vi "leybold.vi"() -> ()   [LabVIEW 2023]
panel:
  in  "RS232":bool
  in  "recipes":bool
  out "Time":timestamp format="%<%H:%M:%S\n%x>T"
  out "Timer end":timestamp format="%<%H:%M:%S>T"
  in  "P3":bool
  in  "P2":bool
  in  "Presets":bool
  out "PR4000":string
  in  "TimerOn":bool
  in  "Matchbox mode":bool
  in  "Timer":bool
  in  "GAS Boost":bool
  in  "-100":bool
  in  "-10":bool
  in  "-1":bool
  in  "+1":bool
  in  "+10":bool
  in  "Gas":bool
  in  "O2 (SCCM)":bool
  in  "Ar (SCCM)":bool
  out "DC Bias (V)":i16
  in  "+100":bool
  in  "Stop":bool
  out "read buffer":string
  out "PFG600":string
  in  "RF Source":bool
  in  "CT":bool
  in  "CL":bool
  in  "FWD Power (W)":bool=TRUE
  out "REF Power (W)":i16
  # "GENERATOR"
  # "MFC"
  # "TIMER"
  # "DEBUG"
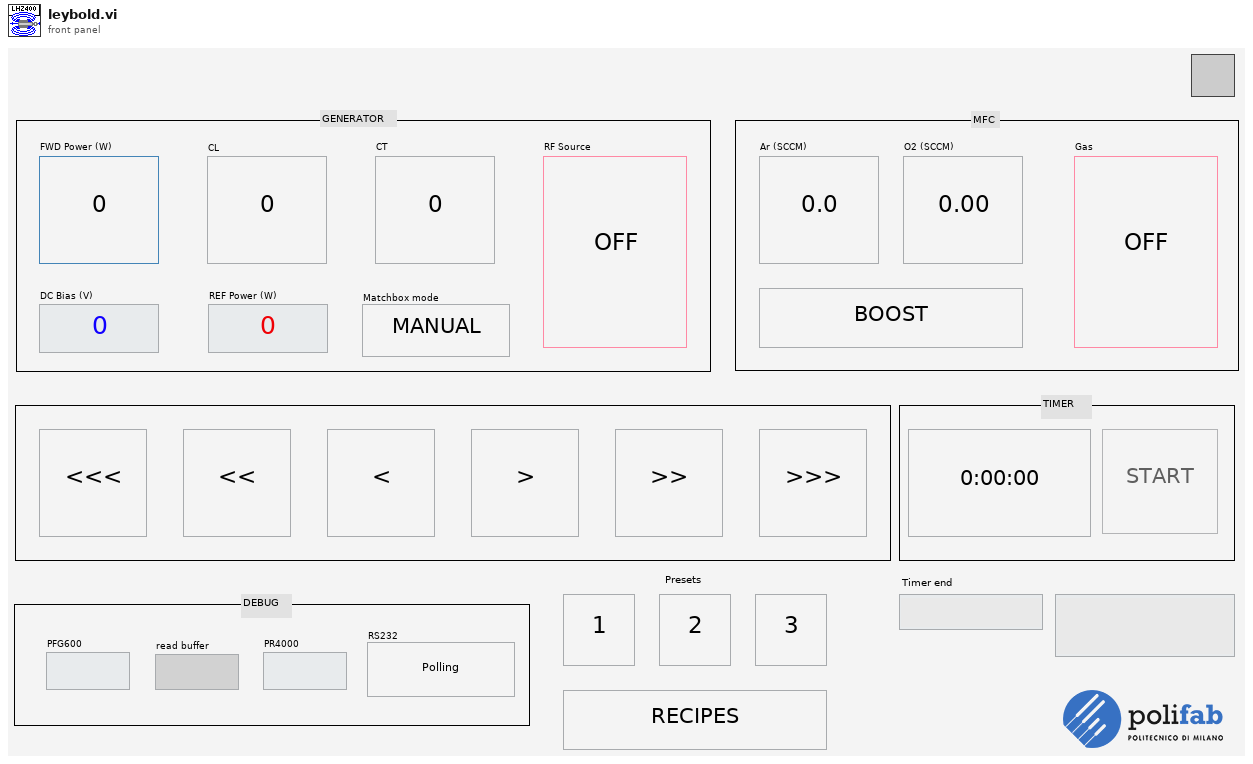
[diagram p1: front panel]
types:
  T1 = enum8{"Enabled", "Disabled", "Disabled and Grayed Out"}
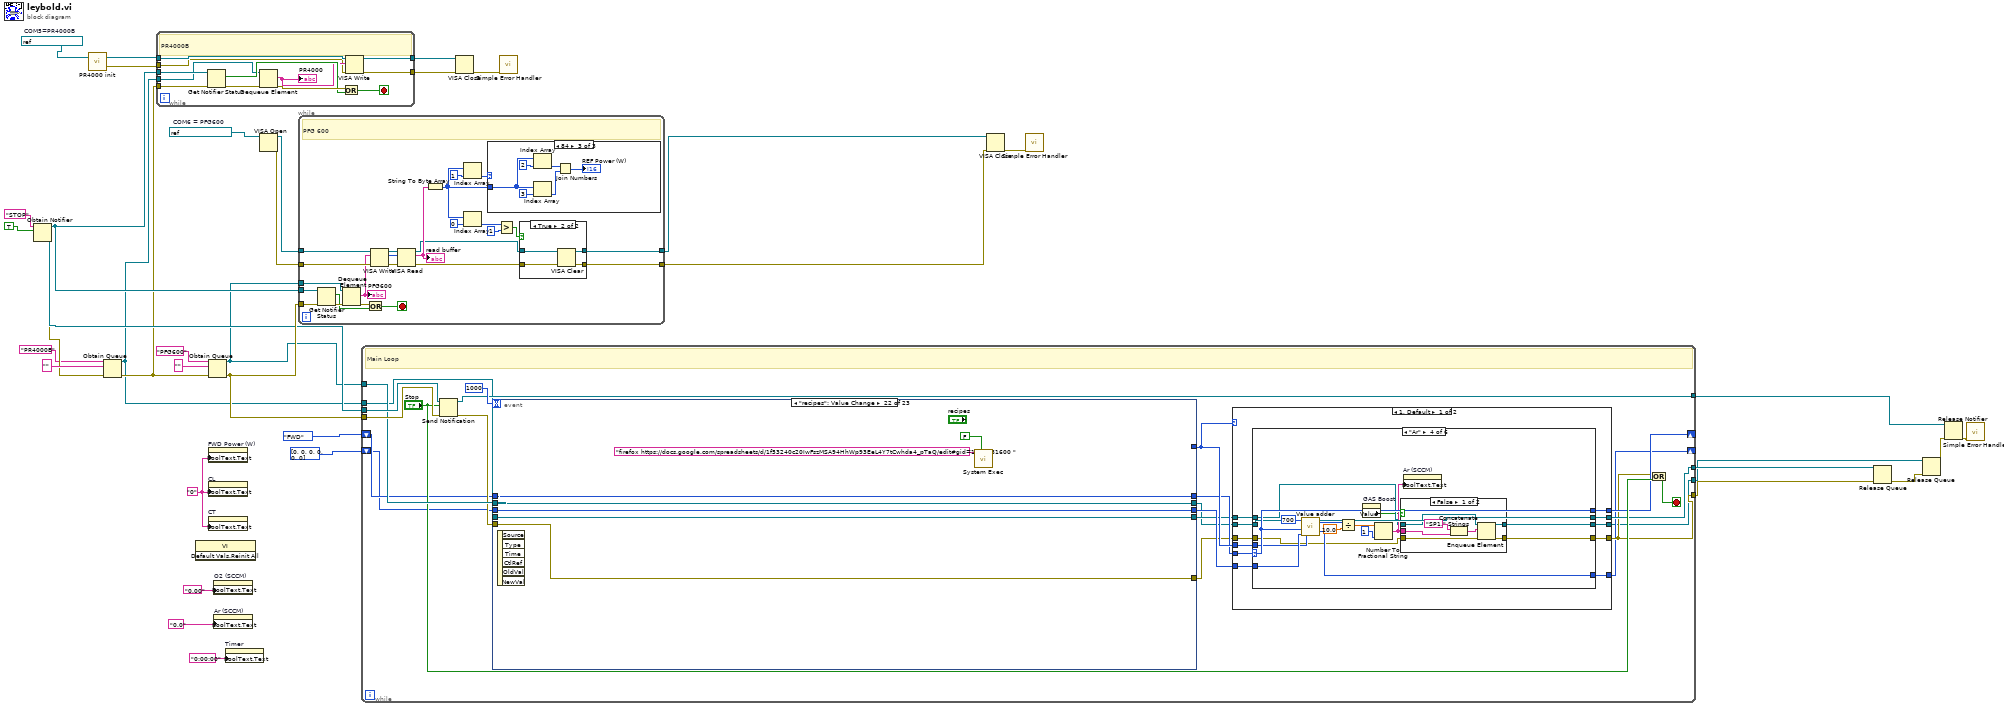
[diagram p0: block diagram]
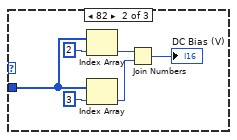
[diagram p4: hidden frame]
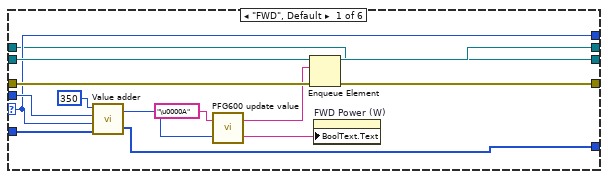
[diagram p5: hidden frame]
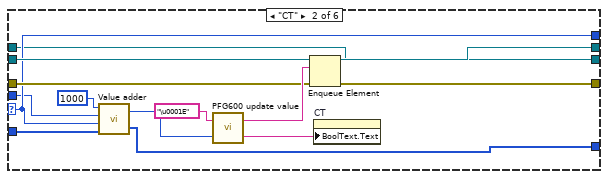
[diagram p6: hidden frame]
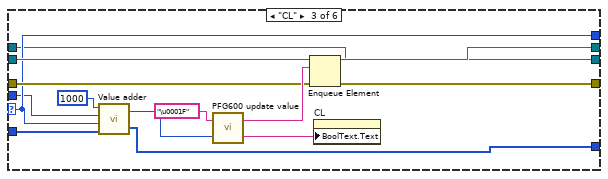
[diagram p7: hidden frame]
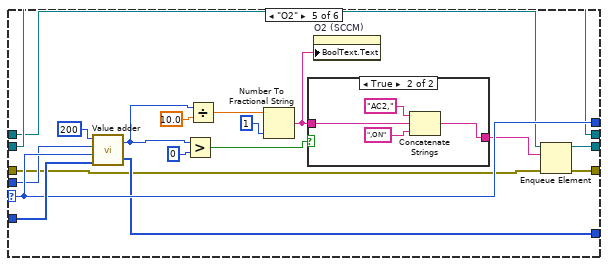
[diagram p9: hidden frame]
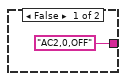
[diagram p10: hidden frame]
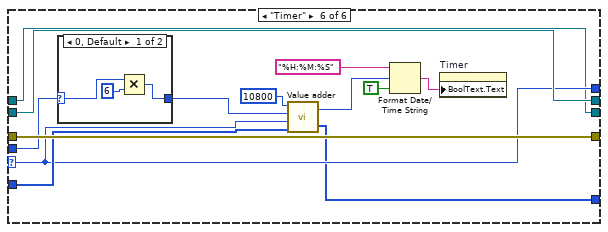
[diagram p11: hidden frame]
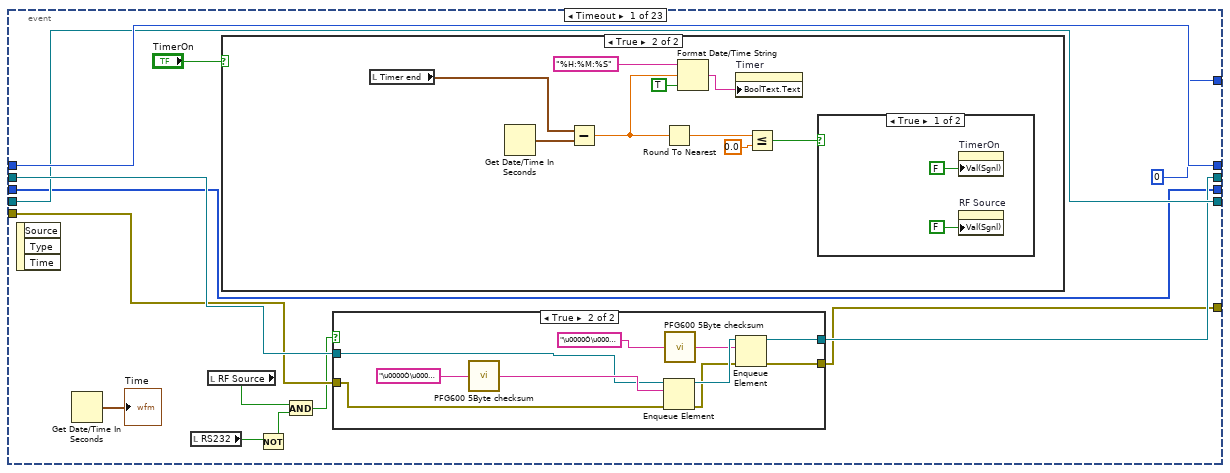
[diagram p14: hidden frame]
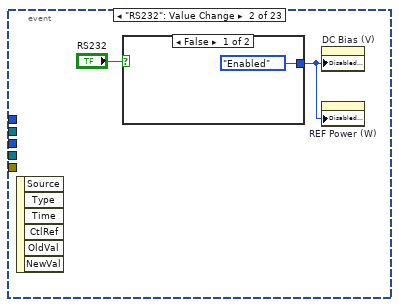
[diagram p18: hidden frame]
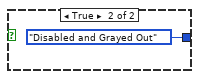
[diagram p19: hidden frame]
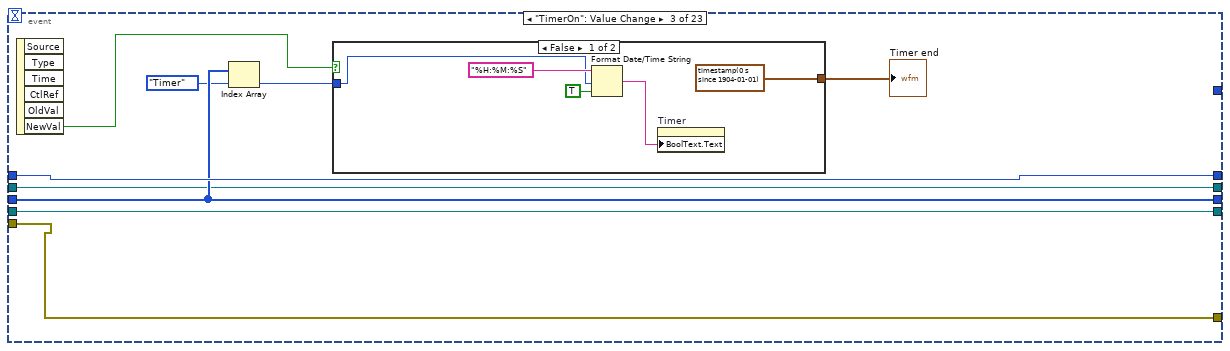
[diagram p20: hidden frame]
diagram:
  w15 = "0" ("Boolean Text.Text")
  w4 = refnum<visa-resource-name> "ASRL33::INSTR"  # COM5=PR4000B
  w37 = refnum<visa-resource-name> "ASRL34::INSTR"  # COM6 = PFG600
  n1 = Obtain Notifier(name (unnamed)="STOP", notification data type=TRUE) -> (notifier out=w22:refnum<notifier>, error out=w11:errorcluster)  [unwired: 2 in, 1 out]
  n2 = call "PR4000 init.vi"("VISA Refnum in"=w4) -> ("error out"=w2:errorcluster, "VISA Refnum out"=w3:refnum<visa-resource-name>)  [unwired: 1 in]
  n3 = Obtain Queue(name (unnamed)="PR4000B", element data type="", error in (no error)=w11) -> (queue out=w17:refnum<queue>, error out=w21:errorcluster)  [unwired: 2 in, 1 out]
  n4 = while {
    tunnel: w3 -> [w45]
    tunnel: w22 -> [w44]
    tunnel: w21 -> [w40]
    tunnel: w17 -> [w43]
    tunnel: [w42] -> w19
    tunnel: [w41] -> w18
    tunnel: w2 -> [w38]
    stop <- w47 stop-if-true
    # "PR4000B"
    n5 = Get Notifier Status(notifier=w44, error in (no error)=w40) -> (current notification=w48:bool, error out=w39:errorcluster)  [unwired: 3 out]
    n6 = Dequeue Element(queue=w43, error in (no error)=w39) -> (element=w46:string, error out=w49:errorcluster)  [unwired: 1 in, 2 out]
    "PR4000" <- w46
    n7 = Or(x=w49, y=w48) -> (x .or. y?=w47:bool)
    n8 = VISA Write(VISA resource name=w45, write buffer=w46, error in (no error)=w38) -> (VISA resource name out=w41:refnum<visa-resource-name>, error out=w42:errorcluster)  [unwired: 1 out]
  }
  n9 = invoke class="VI" method="Default Vals.Reinit All"() -> ()  [unwired: 3 in, 3 out]
  n10 = Obtain Queue(name (unnamed)="PFG600", element data type="", error in (no error)=w21) -> (queue out=w6:refnum<queue>, error out=w30:errorcluster)  [unwired: 2 in, 1 out]
  n11 = property on="FWD Power (W)" class="Bool (strict)"("BoolText.Text"=w15) -> ()  [unwired: 2 in, 2 out]
  n12 = property on="CL" class="Bool (strict)"("BoolText.Text"=w15) -> ()  [unwired: 2 in, 2 out]
  n13 = property on="CT" class="Bool (strict)"("BoolText.Text"=w15) -> ()  [unwired: 2 in, 2 out]
  n14 = property on="O2 (SCCM)" class="Bool (strict)"("BoolText.Text"="0.00") -> ()  [unwired: 2 in, 2 out]
  n15 = property on="Ar (SCCM)" class="Bool (strict)"("BoolText.Text"="0.0") -> ()  [unwired: 2 in, 2 out]
  n16 = property on="Timer" class="Bool (strict)"("BoolText.Text"="0:00:00" ("Boolean Text.Text")) -> ()  [unwired: 2 in, 2 out]
  n17 = VISA Open(VISA resource name=w37) -> (VISA resource name=w28:refnum<visa-resource-name>, error out=w29:errorcluster)  [unwired: 4 in]
  n18 = while {
    tunnel: w22 -> [w73]
    tunnel: w30 -> [w74]
    tunnel: w6 -> [w71]
    tunnel: w29 -> [w65]
    tunnel: w28 -> [w64]
    tunnel: [w50] -> w27
    tunnel: [w51] -> w26
    stop <- w68 stop-if-true
    # "PFG 600"
    n19 = Get Notifier Status(notifier=w73, error in (no error)=w74) -> (current notification=w69:bool, error out=w72:errorcluster)  [unwired: 3 out]
    n20 = Dequeue Element(queue=w71, error in (no error)=w72) -> (element=w63:string, error out=w70:errorcluster)  [unwired: 1 in, 2 out]
    "PFG600" <- w63
    n21 = Or(x=w70, y=w69) -> (x .or. y?=w68:bool)
    n22 = VISA Write(VISA resource name=w64, write buffer=w63, error in (no error)=w65) -> (VISA resource name out=w67:refnum<visa-resource-name>, return count=w59:u32, error out=w66:errorcluster)
    n23 = VISA Read(VISA resource name=w67, byte count=w59, error in (no error)=w66) -> (VISA resource name out=w53:refnum<visa-resource-name>, read buffer=w62:string, error out=w52:errorcluster)  [unwired: 1 out]
    "read buffer" <- w62
    n24 = String To Byte Array(string=w62) -> (unsigned byte array=w58:u8[])
    n25 = Index Array(array=w58, index=1) -> (element=w60:u8)
    n26 = Index Array(array=w58, index=0) -> (element=w56:u8)
    n27 = case shown="84" w60 {
      tunnel: w58 -> [_ w82 w88]
      frame Default {
      }
      frame 82 {
        n28 = Index Array(array=w82, index=2) -> (element=w86:u8)
        n29 = Index Array(array=w82, index=3) -> (element=w84:u8)
        n30 = Join Numbers(hi=w86, lo=w84) -> ((hi.lo)=→"DC Bias (V)":u16)
      }
      frame 84 {
        n31 = Index Array(array=w88, index=2) -> (element=w92:u8)
        n32 = Index Array(array=w88, index=3) -> (element=w90:u8)
        n33 = Join Numbers(hi=w92, lo=w90) -> ((hi.lo)=→"REF Power (W)":u16)
      }
    }
    n34 = Greater?(x=w56, y=u8 1) -> (0:w54:bool)
    n35 = case shown="True" w54 {
      tunnel: w53 -> [w76 w80]
      tunnel: w52 -> [w75 w79]
      tunnel: [w75 w78] -> w50
      tunnel: [w76 w77] -> w51
      frame False {
      }
      frame True {
        n36 = VISA Clear(VISA resource name=w80, error in (no error)=w79) -> (VISA resource name out=w77:refnum<visa-resource-name>, error out=w78:errorcluster)
      }
    }
  }
  n37 = while {
    tunnel: w22 -> [w114]
    tunnel: w30 -> [w113]
    tunnel: [w108] -> w32
    tunnel: w6 -> [w110]
    tunnel: [w105] -> w33
    tunnel: [w104] -> w34
    shift-right: [w106] -> _
    shift-left: enum16{"FWD", "CL", "CT", "Ar", "O2", "Timer"}."FWD" -> [w102]
    shift-right: [w98] -> _
    shift-left: i16[] [0, 0, 0, 0, 0, 0] -> [w100]
    tunnel: w17 -> [w97]
    tunnel: [w94] -> w5
    stop <- w112 stop-if-true
    # "Main Loop"
    n38 = Send Notification(notification="Stop", notifier=w114, error in (no error)=w113) -> (notifier out=w108:refnum<notifier>, error out=w107:errorcluster)
    n39 = event shown="[21] \"recipes\": Value Change" {
      selector: _ -> [_ _ _ _ _ _ _ _ _ _ _ _ _ _ _ _ _ _ _ _ _ _ _]
      dyn-events: _ -> [_ _ _ _ _ _ _ _ _ _ _ _ _ _ _ _ _ _ _ _ _ _ _]
      timeout: u32 1000 ("milliseconds to wait") -> [_ _ _ _ _ _ _ _ _ _ _ _ _ _ _ _ _ _ _ _ _ _ _]
      tunnel: w110 -> [w248 _ w280 w298 w303 w309 w316 w321 w328 w333 w340 w347 w355 w361 w369 w395 w418 w441 w448 w460 w477 w491 w501]
      tunnel: w107 -> [w244 _ w281 w297 w302 w310 w315 w320 w327 w332 w339 w348 w354 w360 w368 w379 w402 w425 w449 _ w478 w488 w502]
      tunnel: [w251 _ w287 w300 w306 w312 w318 w324 w330 enum16{"FWD", "CL", "CT", "Ar", "O2", "Timer"}."CL" enum16{"FWD", "CL", "CT", "Ar", "O2", "Timer"}."FWD" enum16{"FWD", "CL", "CT", "Ar", "O2", "Timer"}."CT" enum16{"FWD", "CL", "CT", "Ar", "O2", "Timer"}."Ar" enum16{"FWD", "CL", "CT", "Ar", "O2", "Timer"}."O2" enum16{"FWD", "CL", "CT", "Ar", "O2", "Timer"}."Timer" w396 w419 w442 w447 w466 w485 w492 w500] -> w101
      tunnel: [0 _ _ 1 -1 10 -10 100 -100 _ _ _ _ _ _ _ _ _ _ _ _ _ _] -> w103
      tunnel: w102 -> [w251 _ w287 w300 w306 w312 w318 w324 w330 _ _ _ _ _ _ w396 w419 w442 w447 w466 w485 w492 w500]
      tunnel: w100 -> [w242 _ w286 w299 w305 w311 w317 w323 w329 w335 w342 w349 w356 w363 w370 w389 w412 w435 w446 w462 w481 w490 w495]
      tunnel: w97 -> [w246 _ w279 w296 w304 w308 w314 w322 w326 w334 w341 w346 w353 w362 w367 w374 w397 w420 w444 w464 w482 w489 w498]
      tunnel: [w242 _ w286 w299 w305 w311 w317 w323 w329 w335 w342 w349 w356 w363 w370 w383 w406 w429 w446 w462 w481 w490 w495] -> w99
      tunnel: [w246 _ w279 w296 w304 w308 w314 w322 w326 w334 w341 w346 w353 w362 w367 w374 w397 w420 w444 w461 w480 w489 w498] -> w96
      tunnel: [w245 _ w280 w298 w303 w309 w316 w321 w328 w333 w340 w347 w355 w361 w369 w375 w398 w421 w445 w460 w477 w491 w497] -> w95
      tunnel: [w243 _ w281 w297 w302 w310 w315 w320 w327 w332 w339 w348 w354 w360 w368 w376 w399 w422 w443 w459 w479 w488 w496] -> w93
      event Timeout {
        n40 = event-data() -> ()  [unwired: 1 in, 3 out]
        n41 = Get Date/Time In Seconds() -> (seconds since 1Jan1904=→"Time":timestamp)
        n42 = local read "RS232"() -> (w238:bool)
        n43 = local read "RF Source"() -> (w240:bool)
        n44 = case shown="True" "TimerOn" {
          frame False {
          }
          frame True {
            n45 = local read "Timer end"() -> (w272:timestamp)
            n46 = Get Date/Time In Seconds() -> (seconds since 1Jan1904=w271:timestamp)
            n47 = Subtract(x=w272, y=w271) -> (x-y=w264:dbl)
            n48 = Round To Nearest(number=w264) -> (nearest integer value=w270:dbl)
            n49 = Format Date/Time String(time format string (%c)="%H:%M:%S", seconds (now)=w264, UTC format=TRUE) -> (date/time string=w265:string)
            n50 = property on="Timer" class="Bool (strict)"("BoolText.Text"=w265) -> ()  [unwired: 2 in, 2 out]
            n51 = Less Or Equal?(x=w270, y=0.0) -> (x <= y?=w268:bool)
            n52 = case shown="True" w268 {
              frame True {
                n53 = property on="TimerOn" class="Bool (strict)"("Val(Sgnl)"=FALSE ("Value (Signaling)")) -> ()  [unwired: 2 in, 2 out]
                n54 = property on="RF Source" class="Bool (strict)"("Val(Sgnl)"=FALSE ("RF Source")) -> ()  [unwired: 2 in, 2 out]
              }
              frame False {
              }
            }
          }
        }
        n55 = Not(x=w238) -> (.not. x?=w239:bool)
        n56 = And(x=w240, y=w239) -> (x .and. y?=w241:bool)
        n57 = case shown="True" w241 {
          tunnel: w248 -> [w253 w258]
          tunnel: [w253 w257] -> w245
          tunnel: w244 -> [w252 w256]
          tunnel: [w252 w254] -> w243
          frame False {
          }
          frame True {
            n58 = call "PFG600 5Byte checksum.vi"("Input"="\u0000Ò\u0000\u0000") -> ("Output"=w263:string)
            n59 = Enqueue Element(queue=w258, element=w263, error in (no error)=w256) -> (queue out=w261:refnum<queue>, error out=w255:errorcluster)  [unwired: 1 in, 1 out]
            n60 = call "PFG600 5Byte checksum.vi"("Input"="\u0000Ô\u0000\u0000") -> ("Output"=w260:string)
            n61 = Enqueue Element(queue=w261, element=w260, error in (no error)=w255) -> (queue out=w257:refnum<queue>, error out=w254:errorcluster)  [unwired: 1 in, 1 out]
          }
        }
      }
      event "RS232": Value Change {
        n62 = event-data() -> ()  [unwired: 1 in, 6 out]
        n63 = case shown="False" "RS232" {
          tunnel: [T1."Enabled" ("Disabled") T1."Disabled and Grayed Out" ("Disabled")] -> w276
          frame False {
          }
          frame True {
          }
        }
        n64 = property on="DC Bias (V)" class="DigNum (strict)"("DisabledEnum"=w276) -> ()  [unwired: 2 in, 2 out]
        n65 = property on="REF Power (W)" class="DigNum (strict)"("DisabledEnum"=w276) -> ()  [unwired: 2 in, 2 out]
      }
      event "TimerOn": Value Change {
        n66 = event-data() -> ("NewVal"=w284:bool)  [unwired: 1 in, 5 out]
        n67 = Index Array(array=w286, index=enum16{"FWD", "CL", "CT", "Ar", "O2", "Timer"}."Timer") -> (element=w283:i16)
        n68 = case shown="False" w284 {
          tunnel: w283 -> [w289 w294]
          tunnel: [timestamp(0 s since 1904-01-01) w293] -> w282
          frame False {
            n69 = Format Date/Time String(time format string (%c)="%H:%M:%S", seconds (now)=w289, UTC format=TRUE) -> (date/time string=w288:string)
            n70 = property on="Timer" class="Bool (strict)"("BoolText.Text"=w288) -> ()  [unwired: 2 in, 2 out]
          }
          frame True {
            n71 = Get Date/Time In Seconds() -> (seconds since 1Jan1904=w295:timestamp)
            n72 = Add(x=w295, y=w294) -> (x+y=w293:timestamp)
          }
        }
        "Timer end" <- w282
      }
      event "+1": Value Change {
        n73 = event-data() -> ()  [unwired: 1 in, 3 out]
      }
      event "-1": Value Change {
        n74 = event-data() -> ()  [unwired: 1 in, 6 out]
      }
      event "+10": Value Change {
        n75 = event-data() -> ()  [unwired: 1 in, 6 out]
      }
      event "-10": Value Change {
        n76 = event-data() -> ()  [unwired: 1 in, 6 out]
      }
      event "+100": Value Change {
        n77 = event-data() -> ()  [unwired: 1 in, 6 out]
      }
      event "-100": Value Change {
        n78 = event-data() -> ()  [unwired: 1 in, 6 out]
      }
      event "CL": Value Change {
        w336 = FALSE ("FWD Power (W)")
        n79 = event-data() -> ()  [unwired: 1 in, 6 out]
        n80 = property on="CL" class="Bool (strict)"("Value"=TRUE ("CL")) -> ()  [unwired: 2 in, 2 out]
        n81 = property on="CT" class="Bool (strict)"("Value"=w336) -> ()  [unwired: 2 in, 2 out]
        n82 = property on="Ar (SCCM)" class="Bool (strict)"("Value"=w336) -> ()  [unwired: 2 in, 2 out]
        n83 = property on="Timer" class="Bool (strict)"("Value"=w336) -> ()  [unwired: 2 in, 2 out]
        n84 = property on="O2 (SCCM)" class="Bool (strict)"("Value"=w336) -> ()  [unwired: 2 in, 2 out]
        n85 = property on="FWD Power (W)" class="Bool (strict)"("Value"=w336) -> ()  [unwired: 2 in, 2 out]
      }
      event "FWD Power (W)": Value Change {
        w343 = FALSE ("FWD Power (W)")
        n86 = event-data() -> ()  [unwired: 1 in, 6 out]
        n87 = property on="FWD Power (W)" class="Bool (strict)"("Value"=TRUE ("CL")) -> ()  [unwired: 2 in, 2 out]
        n88 = property on="CT" class="Bool (strict)"("Value"=w343) -> ()  [unwired: 2 in, 2 out]
        n89 = property on="Ar (SCCM)" class="Bool (strict)"("Value"=w343) -> ()  [unwired: 2 in, 2 out]
        n90 = property on="Timer" class="Bool (strict)"("Value"=w343) -> ()  [unwired: 2 in, 2 out]
        n91 = property on="CL" class="Bool (strict)"("Value"=w343) -> ()  [unwired: 2 in, 2 out]
        n92 = property on="O2 (SCCM)" class="Bool (strict)"("Value"=w343) -> ()  [unwired: 2 in, 2 out]
      }
      event "CT": Value Change {
        w351 = FALSE ("FWD Power (W)")
        n93 = event-data() -> ()  [unwired: 1 in, 6 out]
        n94 = property on="CT" class="Bool (strict)"("Value"=TRUE ("CL")) -> ()  [unwired: 2 in, 2 out]
        n95 = property on="CL" class="Bool (strict)"("Value"=w351) -> ()  [unwired: 2 in, 2 out]
        n96 = property on="Ar (SCCM)" class="Bool (strict)"("Value"=w351) -> ()  [unwired: 2 in, 2 out]
        n97 = property on="Timer" class="Bool (strict)"("Value"=w351) -> ()  [unwired: 2 in, 2 out]
        n98 = property on="O2 (SCCM)" class="Bool (strict)"("Value"=w351) -> ()  [unwired: 2 in, 2 out]
        n99 = property on="FWD Power (W)" class="Bool (strict)"("Value"=w351) -> ()  [unwired: 2 in, 2 out]
      }
      event "Ar (SCCM)": Value Change {
        w357 = FALSE ("FWD Power (W)")
        n100 = event-data() -> ()  [unwired: 1 in, 6 out]
        n101 = property on="Ar (SCCM)" class="Bool (strict)"("Value"=TRUE ("CL")) -> ()  [unwired: 2 in, 2 out]
        n102 = property on="CL" class="Bool (strict)"("Value"=w357) -> ()  [unwired: 2 in, 2 out]
        n103 = property on="CT" class="Bool (strict)"("Value"=w357) -> ()  [unwired: 2 in, 2 out]
        n104 = property on="Timer" class="Bool (strict)"("Value"=w357) -> ()  [unwired: 2 in, 2 out]
        n105 = property on="O2 (SCCM)" class="Bool (strict)"("Value"=w357) -> ()  [unwired: 2 in, 2 out]
        n106 = property on="FWD Power (W)" class="Bool (strict)"("Value"=w357) -> ()  [unwired: 2 in, 2 out]
      }
      event "O2 (SCCM)": Value Change {
        w365 = FALSE ("FWD Power (W)")
        n107 = event-data() -> ()  [unwired: 1 in, 6 out]
        n108 = property on="O2 (SCCM)" class="Bool (strict)"("Value"=TRUE ("CL")) -> ()  [unwired: 2 in, 2 out]
        n109 = property on="CL" class="Bool (strict)"("Value"=w365) -> ()  [unwired: 2 in, 2 out]
        n110 = property on="CT" class="Bool (strict)"("Value"=w365) -> ()  [unwired: 2 in, 2 out]
        n111 = property on="Ar (SCCM)" class="Bool (strict)"("Value"=w365) -> ()  [unwired: 2 in, 2 out]
        n112 = property on="Timer" class="Bool (strict)"("Value"=w365) -> ()  [unwired: 2 in, 2 out]
        n113 = property on="FWD Power (W)" class="Bool (strict)"("Value"=w365) -> ()  [unwired: 2 in, 2 out]
      }
      event "Timer": Value Change {
        w371 = FALSE ("FWD Power (W)")
        n114 = event-data() -> ()  [unwired: 1 in, 6 out]
        n115 = property on="Timer" class="Bool (strict)"("Value"=TRUE ("CL")) -> ()  [unwired: 2 in, 2 out]
        n116 = property on="CL" class="Bool (strict)"("Value"=w371) -> ()  [unwired: 2 in, 2 out]
        n117 = property on="CT" class="Bool (strict)"("Value"=w371) -> ()  [unwired: 2 in, 2 out]
        n118 = property on="Ar (SCCM)" class="Bool (strict)"("Value"=w371) -> ()  [unwired: 2 in, 2 out]
        n119 = property on="FWD Power (W)" class="Bool (strict)"("Value"=w371) -> ()  [unwired: 2 in, 2 out]
        n120 = property on="O2 (SCCM)" class="Bool (strict)"("Value"=w371) -> ()  [unwired: 2 in, 2 out]
      }
      event "Presets": Value Change {
        n121 = event-data() -> ()  [unwired: 1 in, 6 out]
        n122 = call "Value setter.vi"("Array"=w389, "Enum"=enum16{"FWD", "CL", "CT", "Ar", "O2", "Timer"}."CT", "value"=0) -> ("output array"=w384:i16[], "value"=w388:i16)  [unwired: 1 in]
        n123 = call "PFG600 update value.vi"("Value"=w388, "Command"="\u0001E") -> ("Text"=w380:string, "Hex"=w392:string)
        n124 = call "Value setter.vi"("Array"=w384, "Enum"=enum16{"FWD", "CL", "CT", "Ar", "O2", "Timer"}."CL", "value"=1000) -> ("output array"=w383:i16[], "value"=w387:i16)  [unwired: 1 in]
        n125 = property on="CT" class="Bool (strict)"("BoolText.Text"=w380) -> ()  [unwired: 2 in, 2 out]
        n126 = Enqueue Element(queue=w395, element=w392, error in (no error)=w379) -> (queue out=w394:refnum<queue>, error out=w378:errorcluster)  [unwired: 1 in, 1 out]
        n127 = call "PFG600 update value.vi"("Value"=w387, "Command"="\u0001F") -> ("Text"=w381:string, "Hex"=w382:string)
        n128 = property on="CL" class="Bool (strict)"("BoolText.Text"=w381) -> ()  [unwired: 2 in, 2 out]
        n129 = Enqueue Element(queue=w394, element=w382, error in (no error)=w378) -> (queue out=w375:refnum<queue>, error out=w376:errorcluster)  [unwired: 1 in, 1 out]
      }
      event "P2": Value Change {
        n130 = event-data() -> ()  [unwired: 1 in, 6 out]
        n131 = call "Value setter.vi"("Array"=w412, "Enum"=enum16{"FWD", "CL", "CT", "Ar", "O2", "Timer"}."CT", "value"=750) -> ("output array"=w407:i16[], "value"=w411:i16)  [unwired: 1 in]
        n132 = call "PFG600 update value.vi"("Value"=w411, "Command"="\u0001E") -> ("Text"=w403:string, "Hex"=w415:string)
        n133 = call "Value setter.vi"("Array"=w407, "Enum"=enum16{"FWD", "CL", "CT", "Ar", "O2", "Timer"}."CL", "value"=250) -> ("output array"=w406:i16[], "value"=w410:i16)  [unwired: 1 in]
        n134 = property on="CT" class="Bool (strict)"("BoolText.Text"=w403) -> ()  [unwired: 2 in, 2 out]
        n135 = Enqueue Element(queue=w418, element=w415, error in (no error)=w402) -> (queue out=w417:refnum<queue>, error out=w401:errorcluster)  [unwired: 1 in, 1 out]
        n136 = call "PFG600 update value.vi"("Value"=w410, "Command"="\u0001F") -> ("Text"=w404:string, "Hex"=w405:string)
        n137 = property on="CL" class="Bool (strict)"("BoolText.Text"=w404) -> ()  [unwired: 2 in, 2 out]
        n138 = Enqueue Element(queue=w417, element=w405, error in (no error)=w401) -> (queue out=w398:refnum<queue>, error out=w399:errorcluster)  [unwired: 1 in, 1 out]
      }
      event "P3": Value Change {
        n139 = event-data() -> ()  [unwired: 1 in, 6 out]
        n140 = call "Value setter.vi"("Array"=w435, "Enum"=enum16{"FWD", "CL", "CT", "Ar", "O2", "Timer"}."CT", "value"=580) -> ("output array"=w430:i16[], "value"=w434:i16)  [unwired: 1 in]
        n141 = call "PFG600 update value.vi"("Value"=w434, "Command"="\u0001E") -> ("Text"=w426:string, "Hex"=w438:string)
        n142 = call "Value setter.vi"("Array"=w430, "Enum"=enum16{"FWD", "CL", "CT", "Ar", "O2", "Timer"}."CL", "value"=680) -> ("output array"=w429:i16[], "value"=w433:i16)  [unwired: 1 in]
        n143 = property on="CT" class="Bool (strict)"("BoolText.Text"=w426) -> ()  [unwired: 2 in, 2 out]
        n144 = Enqueue Element(queue=w441, element=w438, error in (no error)=w425) -> (queue out=w440:refnum<queue>, error out=w424:errorcluster)  [unwired: 1 in, 1 out]
        n145 = call "PFG600 update value.vi"("Value"=w433, "Command"="\u0001F") -> ("Text"=w427:string, "Hex"=w428:string)
        n146 = property on="CL" class="Bool (strict)"("BoolText.Text"=w427) -> ()  [unwired: 2 in, 2 out]
        n147 = Enqueue Element(queue=w440, element=w428, error in (no error)=w424) -> (queue out=w421:refnum<queue>, error out=w422:errorcluster)  [unwired: 1 in, 1 out]
      }
      event "RF Source": Value Change {
        n148 = event-data() -> ()  [unwired: 1 in, 6 out]
        n149 = case shown="False" "RF Source" {
          tunnel: ["\u0000O\u0000\u0000" "\u0000O\u0000\u0001"] -> w451
          frame False {
            w453 = T1."Enabled" ("Disabled")
            n150 = property on="Presets" class="Bool"("DisabledEnum"=w453) -> ()  [unwired: 2 in, 2 out]
            n151 = property on="P2" class="Bool"("DisabledEnum"=w453) -> ()  [unwired: 2 in, 2 out]
            n152 = property on="P3" class="Bool"("DisabledEnum"=w453) -> ()  [unwired: 2 in, 2 out]
            n153 = property on="TimerOn" class="Bool (strict)"("DisabledEnum"=T1."Disabled and Grayed Out" ("Disabled")) -> ()  [unwired: 2 in, 2 out]
          }
          frame True {
            w456 = T1."Disabled and Grayed Out" ("Disabled")
            n154 = property on="TimerOn" class="Bool (strict)"("DisabledEnum"=T1."Enabled" ("Disabled")) -> ()  [unwired: 2 in, 2 out]
            n155 = property on="Presets" class="Bool"("DisabledEnum"=w456) -> ()  [unwired: 2 in, 2 out]
            n156 = property on="P2" class="Bool"("DisabledEnum"=w456) -> ()  [unwired: 2 in, 2 out]
            n157 = property on="P3" class="Bool"("DisabledEnum"=w456) -> ()  [unwired: 2 in, 2 out]
          }
        }
        n158 = call "PFG600 5Byte checksum.vi"("Input"=w451) -> ("Output"=w450:string)
        n159 = Enqueue Element(queue=w448, element=w450, error in (no error)=w449) -> (queue out=w445:refnum<queue>, error out=w443:errorcluster)  [unwired: 1 in, 1 out]
      }
      event "GAS Boost": Value Change {
        n160 = event-data() -> ()  [unwired: 1 in, 6 out]
        n161 = case shown="True" "GAS Boost" {
          tunnel: [w472 "SP1,60.0"] -> w463
          tunnel: w462 -> [w475 _]
          frame False {
            n162 = Index Array(array=w475, index=enum16{"FWD", "CL", "CT", "Ar", "O2", "Timer"}."Ar") -> (element=w469:i16)
            n163 = Divide(x=w469, y=10.0) -> (x/y=w468:dbl)
            n164 = Number To Fractional String(number=w468, precision (6)=i16 1) -> (F-format string=w470:string)  [unwired: 2 in]
            n165 = Concatenate Strings("SP1," ("string"), w470) -> (w472:string)
          }
          frame True {
          }
        }
        n166 = Enqueue Element(queue=w464, element=w463) -> (queue out=w461:refnum<queue>, error out=w459:errorcluster)  [unwired: 2 in, 1 out]
      }
      event "Gas": Value Change {
        n167 = event-data() -> ()  [unwired: 1 in, 6 out]
        n168 = case shown="True" "Gas" {
          tunnel: ["VL0,OFF" ("string") "VL0,ON" ("string")] -> w483
          frame False {
          }
          frame True {
          }
        }
        n169 = Enqueue Element(queue=w482, element=w483, error in (no error)=w478) -> (queue out=w480:refnum<queue>, error out=w479:errorcluster)  [unwired: 1 in, 1 out]
      }
      event "recipes": Value Change {
        n170 = event-data() -> ()  [unwired: 1 in, 6 out]
        n171 = call <vilib>:"System Exec.vi"("wait until completion? (T)"=FALSE, "command line"="firefox https://docs.google.com/spreadsheets/d/1f53240c20IwFszMSA94HhWp93EeL4Y7tCwhda4_pTaQ/edit#gid=1759381600 ") -> ()  [unwired: 6 in, 4 out]
      }
      event "Matchbox mode": Value Change {
        n172 = event-data() -> ()  [unwired: 1 in, 6 out]
        n173 = case shown="True" "Matchbox mode" {
          tunnel: ["\u0001M\u0000\u0001" "\u0001M\u0000\u0002"] -> w504
          frame False {
          }
          frame True {
          }
        }
        n174 = call "PFG600 5Byte checksum.vi"("Input"=w504) -> ("Output"=w503:string)
        n175 = Enqueue Element(queue=w501, element=w503, error in (no error)=w502) -> (queue out=w497:refnum<queue>, error out=w496:errorcluster)  [unwired: 1 in, 1 out]
      }
    }
    n176 = case shown="1, Default" w103 {
      tunnel: w95 -> [w125 w236]
      tunnel: w93 -> [w124 w237]
      tunnel: w99 -> [w123 w235]
      tunnel: w103 -> [w122 _]
      tunnel: [w121 w234] -> w106
      tunnel: [w120 w235] -> w98
      tunnel: [w119 w236] -> w105
      tunnel: [w118 w237] -> w104
      tunnel: w101 -> [w117 w234]
      tunnel: w96 -> [w116 w233]
      tunnel: [w115 w233] -> w94
      frame 1, Default {
        n177 = case shown="\"Ar\"" w117 {
          selector: w117 -> [w130 w144 w159 w181 w208 w223]
          tunnel: [w130 w144 w159 w181 w208 w223] -> w121
          tunnel: w123 -> [w129 w145 w160 w182 w209 w224]
          tunnel: w122 -> [w131 w143 w158 w180 w207 w221]
          tunnel: [w127 w141 w156 w179 w206 w222] -> w120
          tunnel: w125 -> [w137 w151 w166 w178 w205 w228]
          tunnel: w124 -> [w135 w149 w164 w170 w193 w227]
          tunnel: [w136 w148 w163 w178 w205 w228] -> w119
          tunnel: [w133 w147 w162 w169 w194 w227] -> w118
          tunnel: w116 -> [w126 w140 w154 w172 w196 w216]
          tunnel: [w126 w140 w154 w171 w195 w216] -> w115
          frame "FWD", Default {
            n178 = call "Value adder.vi"("Array"=w129, "Enum"=w130, "value"=w131, "Max Limit"=i16 350) -> ("output array"=w127:i16[], "Limited value"=w128:i16)
            n179 = call "PFG600 update value.vi"("Value"=w128, "Command"="\u0000A") -> ("Text"=w139:string, "Hex"=w134:string)
            n180 = Enqueue Element(queue=w137, element=w134, error in (no error)=w135) -> (queue out=w136:refnum<queue>, error out=w133:errorcluster)  [unwired: 1 in, 1 out]
            n181 = property on="FWD Power (W)" class="Bool (strict)"("BoolText.Text"=w139) -> ()  [unwired: 2 in, 2 out]
          }
          frame "CT" {
            n182 = call "Value adder.vi"("Array"=w145, "Enum"=w144, "value"=w143, "Max Limit"=i16 1000) -> ("output array"=w141:i16[], "Limited value"=w142:i16)
            n183 = call "PFG600 update value.vi"("Value"=w142, "Command"="\u0001E") -> ("Text"=w152:string, "Hex"=w150:string)
            n184 = Enqueue Element(queue=w151, element=w150, error in (no error)=w149) -> (queue out=w148:refnum<queue>, error out=w147:errorcluster)  [unwired: 1 in, 1 out]
            n185 = property on="CT" class="Bool (strict)"("BoolText.Text"=w152) -> ()  [unwired: 2 in, 2 out]
          }
          frame "CL" {
            n186 = call "Value adder.vi"("Array"=w160, "Enum"=w159, "value"=w158, "Max Limit"=i16 1000) -> ("output array"=w156:i16[], "Limited value"=w157:i16)
            n187 = call "PFG600 update value.vi"("Value"=w157, "Command"="\u0001F") -> ("Text"=w155:string, "Hex"=w165:string)
            n188 = Enqueue Element(queue=w166, element=w165, error in (no error)=w164) -> (queue out=w163:refnum<queue>, error out=w162:errorcluster)  [unwired: 1 in, 1 out]
            n189 = property on="CL" class="Bool (strict)"("BoolText.Text"=w155) -> ()  [unwired: 2 in, 2 out]
          }
          frame "Ar" {
            n190 = call "Value adder.vi"("Array"=w182, "Enum"=w181, "value"=w180, "Max Limit"=i16 700) -> ("output array"=w179:i16[], "Limited value"=w176:i16)
            n191 = Divide(x=w176, y=10.0) -> (x/y=w175:dbl)
            n192 = property on="GAS Boost" class="Bool (strict)"() -> ("Value"=w168:bool)  [unwired: 2 in, 2 out]
            n193 = Number To Fractional String(number=w175, precision (6)=i16 1) -> (F-format string=w173:string)  [unwired: 2 in]
            n194 = case shown="False" w168 {
              tunnel: w173 -> [w189 _]
              tunnel: w172 -> [w187 w192]
              tunnel: [w186 w192] -> w171
              tunnel: w170 -> [w185 w191]
              tunnel: [w184 w191] -> w169
              frame False {
                n195 = Concatenate Strings("SP1," ("string"), w189) -> (w188:string)
                n196 = Enqueue Element(queue=w187, element=w188, error in (no error)=w185) -> (queue out=w186:refnum<queue>, error out=w184:errorcluster)  [unwired: 1 in, 1 out]
              }
              frame True {
              }
            }
            n197 = property on="Ar (SCCM)" class="Bool (strict)"("BoolText.Text"=w173) -> ()  [unwired: 2 in, 2 out]
          }
          frame "O2" {
            n198 = call "Value adder.vi"("Array"=w209, "Enum"=w208, "value"=w207, "Max Limit"=i16 200) -> ("output array"=w206:i16[], "Limited value"=w200:i16)
            n199 = Greater?(x=w200, y=i16 0) -> (0:w199:bool)
            n200 = Divide(x=w200, y=10.0) -> (x/y=w203:dbl)
            n201 = Number To Fractional String(number=w203, precision (6)=i16 1) -> (F-format string=w198:string)  [unwired: 2 in]
            n202 = case shown="True" w199 {
              tunnel: ["AC2,0,OFF" w212] -> w197
              tunnel: w198 -> [_ w214]
              frame False {
              }
              frame True {
                n203 = Concatenate Strings("AC2," ("string"), w214, ",ON" ("string")) -> (w212:string)
              }
            }
            n204 = property on="O2 (SCCM)" class="Bool (strict)"("BoolText.Text"=w198) -> ()  [unwired: 2 in, 2 out]
            n205 = Enqueue Element(queue=w196, element=w197, error in (no error)=w193) -> (queue out=w195:refnum<queue>, error out=w194:errorcluster)  [unwired: 1 in, 1 out]
          }
          frame "Timer" {
            n206 = case shown="0, Default" w221 {
              selector: w221 -> [w230 w232]
              tunnel: [w231 w232] -> w225
              frame 0, Default {
                n207 = Multiply(x=w230, y=6) -> (x*y=w231:i32)
              }
              frame -1, 1 {
              }
            }
            n208 = call "Value adder.vi"("Array"=w224, "Enum"=w223, "value"=w225, "Max Limit"=i16 10800) -> ("output array"=w222:i16[], "Limited value"=w220:i16)
            n209 = Format Date/Time String(time format string (%c)="%H:%M:%S", seconds (now)=w220, UTC format=TRUE) -> (date/time string=w219:string)
            n210 = property on="Timer" class="Bool (strict)"("BoolText.Text"=w219) -> ()  [unwired: 2 in, 2 out]
          }
        }
      }
      frame 0 {
      }
    }
    n211 = Or(x=w104, y="Stop") -> (x .or. y?=w112:bool)
  }
  n212 = VISA Close(VISA resource name=w18, error in (no error)=w19) -> (error out=w20:errorcluster)
  n213 = call <vilib>:"Simple Error Handler.vi"("error in (no error)"=w20) -> ()  [unwired: 4 in, 5 out]
  n214 = VISA Close(VISA resource name=w26, error in (no error)=w27) -> (error out=w25:errorcluster)
  n215 = call <vilib>:"Simple Error Handler.vi"("error in (no error)"=w25) -> ()  [unwired: 4 in, 5 out]
  n216 = Release Queue(queue=w33, error in (no error)=w34) -> (error out=w7:errorcluster)  [unwired: 1 in, 2 out]
  n217 = Release Queue(queue=w5, error in (no error)=w7) -> (error out=w8:errorcluster)  [unwired: 1 in, 2 out]
  n218 = Release Notifier(notifier=w32, error in (no error)=w8) -> (error out=w31:errorcluster)  [unwired: 1 in, 2 out]
  n219 = call <vilib>:"Simple Error Handler.vi"("error in (no error)"=w31) -> ()  [unwired: 4 in, 5 out]
